vi "Cycling_No_DAQ_Tasks_All_3_PS_RT.vi"() -> ()   [LabVIEW 2020]
uses:
  <instrlib>/NH Research Regenerative Test Series/Public/Configure/Output Safety.ctl
panel:
  in  "PS error in 7":errorcluster caption="PS error in    (no error)"
  out "PS Visa Out 7":refnum<visa-resource-name>
  out "PS error out 7":errorcluster
  in  "PS error in 6":errorcluster caption="PS error in    (no error)"
  out "PS Visa Out 6":refnum<visa-resource-name>
  out "PS error out 6":errorcluster
  in  "PS error in 5":errorcluster caption="PS error in    (no error)"
  out "PS Visa Out 5":refnum<visa-resource-name>
  out "PS error out 5":errorcluster
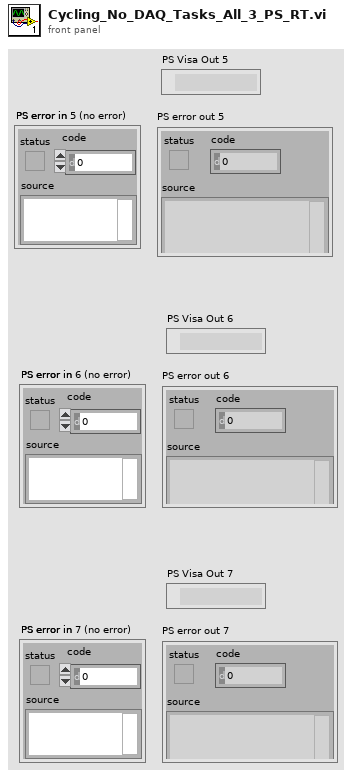
[diagram p1: front panel]
types:
  T1 = enum16{"\"30Q\"", "\"40T\"", "\"2P30Q\"", "\"3P30Q\"", "\"Nissan Leaf\"", ""}
  T2 = typedef "Output Safety.ctl" = cluster{"Min Voltage (V)":dbl, "Min Voltage Time (s)":dbl, "Max Voltage (V)":dbl, "Max Voltage Time (s)":dbl, "Max Sink Current (A)":dbl, "Max Sink Current Time (s)":dbl, "Max Source Current (A)":dbl, "Max Source Current Time (s)":dbl, "Max Sink Power (W)":dbl, "Max Sink Power Time (s)":dbl, "Max Source Power (W)":dbl, "Max Source Power Time (s)":dbl}
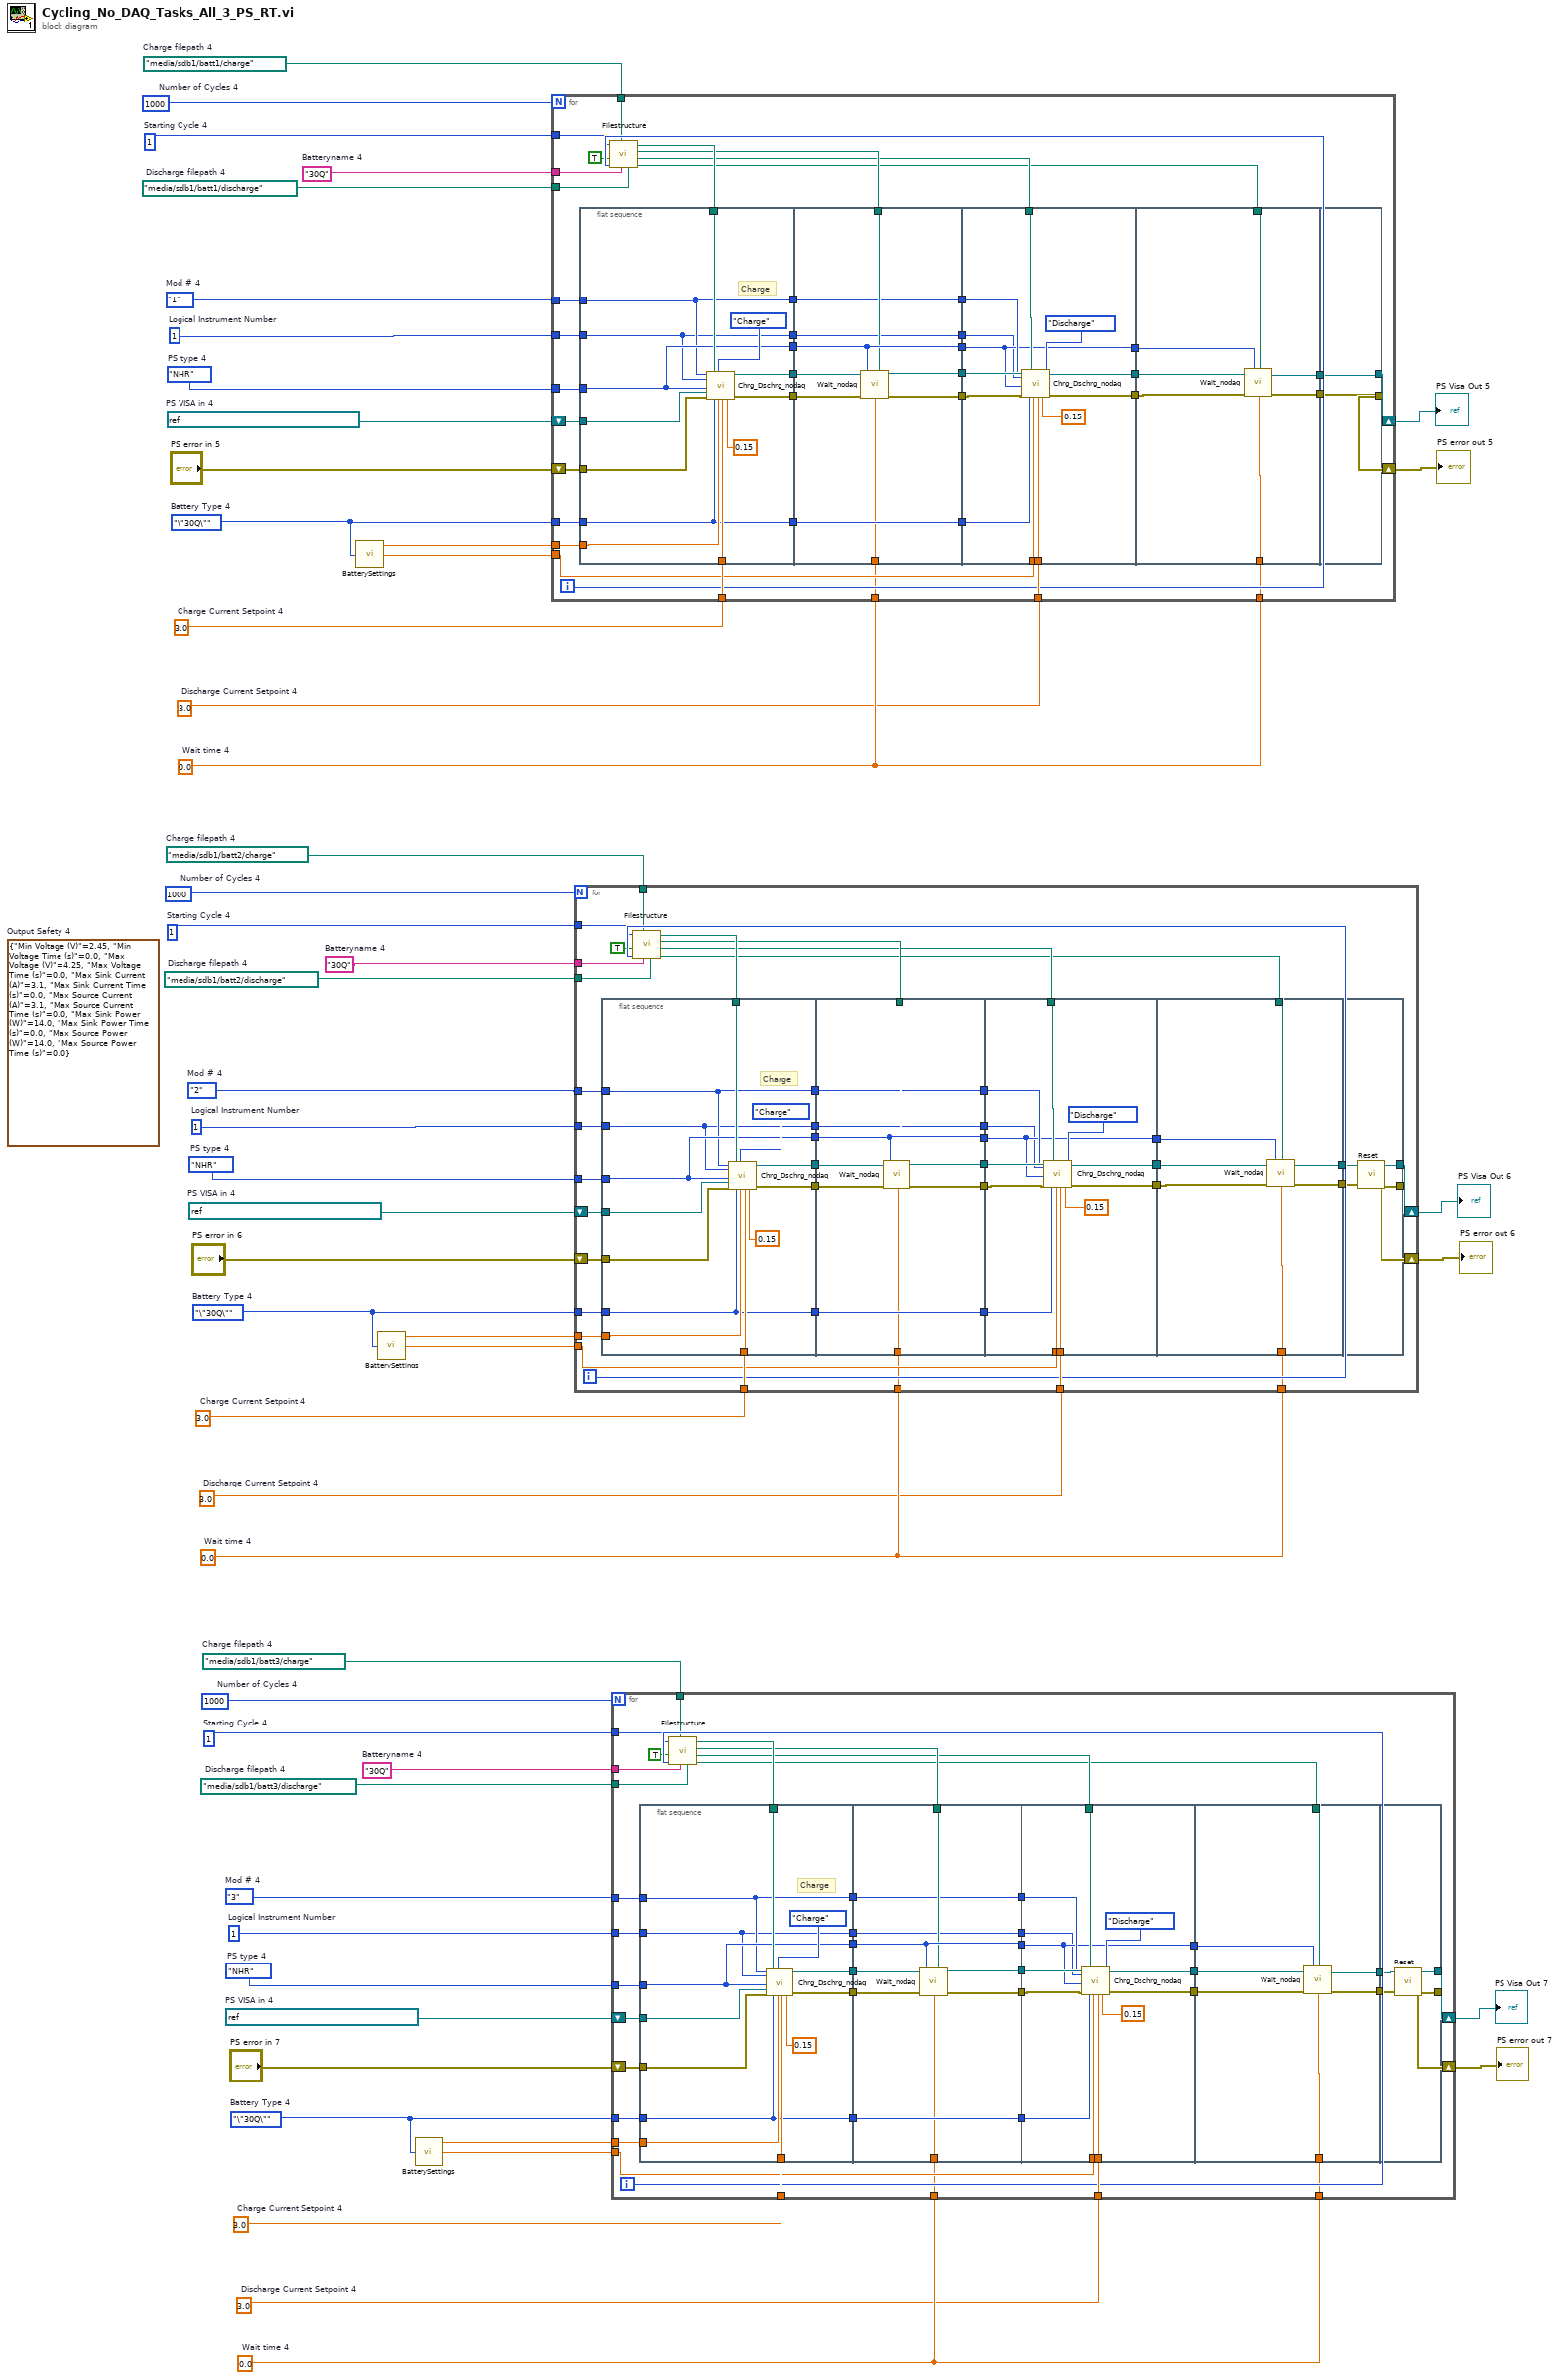
[diagram p0: block diagram]
diagram:
  w1 = u32 1  # Logical Instrument Number
  w3 = 1000  # Number of Cycles 4
  w4 = 1  # Starting Cycle 4
  w2 = path "/media/sdb1/batt3/charge"  # Charge filepath 4
  w5 = "30Q"  # Batteryname 4
  w6 = path "/media/sdb1/batt3/discharge"  # Discharge filepath 4
  w8 = enum16{"ITECH", "NHR"}."NHR"  # PS type 4
  w16 = 0.0  # Wait time 4
  w15 = 3.0  # Discharge Current Setpoint 4
  w14 = 3.0  # Charge Current Setpoint 4
  w11 = T1."\"30Q\""  # Battery Type 4
  w9 = refnum<visa-resource-name> "TCPIP0::192.168.0.94::inst0::INSTR"  # PS VISA in 4
  w7 = enum16{"0", "1", "2", "3"}."3"  # Mod # 4
  w19 = u32 1  # Logical Instrument Number
  w21 = 1000  # Number of Cycles 4
  w22 = 1  # Starting Cycle 4
  w20 = path "/media/sdb1/batt2/charge"  # Charge filepath 4
  w23 = "30Q"  # Batteryname 4
  w24 = path "/media/sdb1/batt2/discharge"  # Discharge filepath 4
  (unwired) T2 {"Min Voltage (V)"=2.45, "Min Voltage Time (s)"=0.0, "Max Voltage (V)"=4.25, "Max Voltage Time (s)"=0.0, "Max Sink Current (A)"=3.1, "Max Sink Current Time (s)"=0.0, "Max Source Current (A)"=3.1, "Max Source Current Time (s)"=0.0, "Max Sink Power (W)"=14.0, "Max Sink Power Time (s)"=0.0, "Max Source Power (W)"=14.0, "Max Source Power Time (s)"=0.0}  # Output Safety 4
  w26 = enum16{"ITECH", "NHR"}."NHR"  # PS type 4
  w34 = 0.0  # Wait time 4
  w33 = 3.0  # Discharge Current Setpoint 4
  w32 = 3.0  # Charge Current Setpoint 4
  w29 = T1."\"30Q\""  # Battery Type 4
  w27 = refnum<visa-resource-name> "TCPIP0::192.168.0.93::inst0::INSTR"  # PS VISA in 4
  w25 = enum16{"0", "1", "2", "3"}."2"  # Mod # 4
  w37 = u32 1  # Logical Instrument Number
  w39 = 1000  # Number of Cycles 4
  w40 = 1  # Starting Cycle 4
  w38 = path "/media/sdb1/batt1/charge"  # Charge filepath 4
  w41 = "30Q"  # Batteryname 4
  w42 = path "/media/sdb1/batt1/discharge"  # Discharge filepath 4
  w44 = enum16{"ITECH", "NHR"}."NHR"  # PS type 4
  w52 = 0.0  # Wait time 4
  w51 = 3.0  # Discharge Current Setpoint 4
  w50 = 3.0  # Charge Current Setpoint 4
  w47 = T1."\"30Q\""  # Battery Type 4
  w45 = refnum<visa-resource-name> "TCPIP0::192.168.0.92::inst0::INSTR"  # PS VISA in 4
  w43 = enum16{"0", "1", "2", "3"}."1"  # Mod # 4
  n1 = call "BatterySettings.vi"("Battery Type"=w47) -> ("Min Voltage (V)"=w49:dbl, "Max Voltage (V)"=w48:dbl)  [unwired: 2 in, 1 out]
  n2 = call "BatterySettings.vi"("Battery Type"=w29) -> ("Min Voltage (V)"=w31:dbl, "Max Voltage (V)"=w30:dbl)  [unwired: 2 in, 1 out]
  n3 = call "BatterySettings.vi"("Battery Type"=w11) -> ("Min Voltage (V)"=w13:dbl, "Max Voltage (V)"=w12:dbl)  [unwired: 2 in, 1 out]
  n4 = for {
    N: w39 -> [_]
    tunnel: w44 -> [w86]
    tunnel: w48 -> [w83]
    tunnel: w47 -> [w82]
    tunnel: w50 -> [w81]
    tunnel: w49 -> [w80]
    tunnel: w51 -> [w79]
    shift-right: [w73] -> w53
    shift-left: w45 -> [w85]
    shift-right: [w74] -> w54
    shift-left: "PS error in 5" -> [w84]
    tunnel: w40 -> [w71]
    tunnel: w41 -> [w69]
    tunnel: w42 -> [w68]
    tunnel: w38 -> [w67]
    tunnel: w52 -> [w62]
    tunnel: w52 -> [w61]
    tunnel: w43 -> [w60]
    tunnel: w37 -> [w57]
    i -> [w72]
    n5 = flat-sequence {
      tunnel: w86 -> [w98]
      tunnel: w85 -> [w100]
      tunnel: w84 -> [w101]
      tunnel: w82 -> [w99]
      tunnel: w83 -> [w102]
      tunnel: w81 -> [w103]
      tunnel: [w98] -> w95
      tunnel: [w99] -> w94
      tunnel: w78 -> [w108]
      tunnel: [w106] -> w64
      tunnel: [w105] -> w63
      tunnel: w60 -> [w97]
      tunnel: [w97] -> w58
      tunnel: w57 -> [w96]
      tunnel: [w96] -> w56
      tunnel: w95 -> [w117]
      tunnel: [w114] -> w93
      tunnel: [w115] -> w92
      tunnel: [w117] -> w91
      tunnel: w94 -> [w118]
      tunnel: [w118] -> w90
      tunnel: w77 -> [w116]
      tunnel: w64 -> [w113]
      tunnel: w63 -> [w112]
      tunnel: w61 -> [w111]
      tunnel: [w110] -> w59
      tunnel: w58 -> [w110]
      tunnel: w56 -> [w109]
      tunnel: [w109] -> w55
      tunnel: w93 -> [w127]
      tunnel: w92 -> [w128]
      tunnel: w91 -> [w121]
      tunnel: w90 -> [w130]
      tunnel: w80 -> [w129]
      tunnel: w79 -> [w120]
      tunnel: w76 -> [w126]
      tunnel: [w123] -> w89
      tunnel: [w124] -> w88
      tunnel: [w121] -> w87
      tunnel: w59 -> [w122]
      tunnel: w55 -> [w119]
      tunnel: w75 -> [w137]
      tunnel: w89 -> [w138]
      tunnel: w88 -> [w135]
      tunnel: w87 -> [w133]
      tunnel: [w136] -> w66
      tunnel: [w134] -> w65
      tunnel: w62 -> [w132]
      tunnel: [w140] -> w73
      tunnel: [w139] -> w74
      tunnel: w66 -> [w139]
      tunnel: w65 -> [w140]
      frame #0 {
        # "Charge"
        n6 = call "Chrg_Dschrg_nodaq.vi"("Mod #"=w97, "Logical Instrument Number"=w96, "PS type"=w98, "PS VISA in"=w100, "PS error in"=w101, "CyclePath"=w108, "Battery Type"=w99, "Charge/discharge"=enum8{"Charge", "Discharge"}."Charge", "Charge/Discharge Voltage Setpoint"=w102, "Current Setpoint"=w103, "Current Cutoff"=0.15) -> ("PS VISA out"=w106:refnum<visa-resource-name>, "PS error out"=w105:errorcluster)  [unwired: 7 in]
      }
      frame #1 {
        n7 = call "Wait_nodaq.vi"("PS type"=w117, "PS VISA in"=w113, "PS error in"=w112, "Wait Filepath"=w116, "Wait time"=w111) -> ("PS Visa Out"=w114:refnum<visa-resource-name>, "PS error out"=w115:errorcluster)  [unwired: 9 in]
      }
      frame #2 {
        n8 = call "Chrg_Dschrg_nodaq.vi"("Mod #"=w122, "Logical Instrument Number"=w119, "PS type"=w121, "PS VISA in"=w127, "PS error in"=w128, "CyclePath"=w126, "Battery Type"=w130, "Charge/discharge"=enum8{"Charge", "Discharge"}."Discharge", "Charge/Discharge Voltage Setpoint"=w129, "Current Setpoint"=w120, "Current Cutoff"=0.15) -> ("PS VISA out"=w123:refnum<visa-resource-name>, "PS error out"=w124:errorcluster)  [unwired: 7 in]
      }
      frame #3 {
        n9 = call "Wait_nodaq.vi"("PS type"=w133, "PS VISA in"=w138, "PS error in"=w135, "Wait Filepath"=w137, "Wait time"=w132) -> ("PS Visa Out"=w134:refnum<visa-resource-name>, "PS error out"=w136:errorcluster)  [unwired: 9 in]
      }
      frame #4 {
      }
    }
    n10 = call "Filestructure.vi"("Discharge filepath"=w68, "Batteryname"=w69, "Charge filepath"=w67, "For loop i"=w72, "In for loop"=TRUE, "Starting Cycle"=w71) -> ("DischargeWaitPath"=w75:path, "DischargeCyclePath"=w76:path, "ChargeWaitPath"=w77:path, "ChargeCyclePath"=w78:path)  [unwired: 1 in, 1 out]
  }
  "PS error out 5" <- w54
  "PS Visa Out 5" <- w53
  n11 = for {
    N: w21 -> [_]
    tunnel: w26 -> [w172]
    tunnel: w30 -> [w169]
    tunnel: w29 -> [w168]
    tunnel: w32 -> [w167]
    tunnel: w31 -> [w166]
    tunnel: w33 -> [w165]
    shift-right: [w159] -> w35
    shift-left: w27 -> [w171]
    shift-right: [w160] -> w36
    shift-left: "PS error in 6" -> [w170]
    tunnel: w22 -> [w157]
    tunnel: w23 -> [w155]
    tunnel: w24 -> [w154]
    tunnel: w20 -> [w153]
    tunnel: w34 -> [w148]
    tunnel: w34 -> [w147]
    tunnel: w25 -> [w146]
    tunnel: w19 -> [w143]
    i -> [w158]
    n12 = flat-sequence {
      tunnel: w172 -> [w184]
      tunnel: w171 -> [w186]
      tunnel: w170 -> [w187]
      tunnel: w168 -> [w185]
      tunnel: w169 -> [w188]
      tunnel: w167 -> [w189]
      tunnel: [w184] -> w181
      tunnel: [w185] -> w180
      tunnel: w164 -> [w194]
      tunnel: [w192] -> w150
      tunnel: [w191] -> w149
      tunnel: w146 -> [w183]
      tunnel: [w183] -> w144
      tunnel: w143 -> [w182]
      tunnel: [w182] -> w142
      tunnel: w181 -> [w203]
      tunnel: [w200] -> w179
      tunnel: [w201] -> w178
      tunnel: [w203] -> w177
      tunnel: w180 -> [w204]
      tunnel: [w204] -> w176
      tunnel: w163 -> [w202]
      tunnel: w150 -> [w199]
      tunnel: w149 -> [w198]
      tunnel: w147 -> [w197]
      tunnel: [w196] -> w145
      tunnel: w144 -> [w196]
      tunnel: w142 -> [w195]
      tunnel: [w195] -> w141
      tunnel: w179 -> [w213]
      tunnel: w178 -> [w214]
      tunnel: w177 -> [w207]
      tunnel: w176 -> [w216]
      tunnel: w166 -> [w215]
      tunnel: w165 -> [w206]
      tunnel: w162 -> [w212]
      tunnel: [w209] -> w175
      tunnel: [w210] -> w174
      tunnel: [w207] -> w173
      tunnel: w145 -> [w208]
      tunnel: w141 -> [w205]
      tunnel: w161 -> [w223]
      tunnel: w175 -> [w224]
      tunnel: w174 -> [w221]
      tunnel: w173 -> [w219]
      tunnel: [w222] -> w152
      tunnel: [w220] -> w151
      tunnel: w148 -> [w218]
      tunnel: [w227] -> w159
      tunnel: [w225] -> w160
      tunnel: w152 -> [w226]
      tunnel: w151 -> [w228]
      frame #0 {
        # "Charge"
        n13 = call "Chrg_Dschrg_nodaq.vi"("Mod #"=w183, "Logical Instrument Number"=w182, "PS type"=w184, "PS VISA in"=w186, "PS error in"=w187, "CyclePath"=w194, "Battery Type"=w185, "Charge/discharge"=enum8{"Charge", "Discharge"}."Charge", "Charge/Discharge Voltage Setpoint"=w188, "Current Setpoint"=w189, "Current Cutoff"=0.15) -> ("PS VISA out"=w192:refnum<visa-resource-name>, "PS error out"=w191:errorcluster)  [unwired: 7 in]
      }
      frame #1 {
        n14 = call "Wait_nodaq.vi"("PS type"=w203, "PS VISA in"=w199, "PS error in"=w198, "Wait Filepath"=w202, "Wait time"=w197) -> ("PS Visa Out"=w200:refnum<visa-resource-name>, "PS error out"=w201:errorcluster)  [unwired: 9 in]
      }
      frame #2 {
        n15 = call "Chrg_Dschrg_nodaq.vi"("Mod #"=w208, "Logical Instrument Number"=w205, "PS type"=w207, "PS VISA in"=w213, "PS error in"=w214, "CyclePath"=w212, "Battery Type"=w216, "Charge/discharge"=enum8{"Charge", "Discharge"}."Discharge", "Charge/Discharge Voltage Setpoint"=w215, "Current Setpoint"=w206, "Current Cutoff"=0.15) -> ("PS VISA out"=w209:refnum<visa-resource-name>, "PS error out"=w210:errorcluster)  [unwired: 7 in]
      }
      frame #3 {
        n16 = call "Wait_nodaq.vi"("PS type"=w219, "PS VISA in"=w224, "PS error in"=w221, "Wait Filepath"=w223, "Wait time"=w218) -> ("PS Visa Out"=w220:refnum<visa-resource-name>, "PS error out"=w222:errorcluster)  [unwired: 9 in]
      }
      frame #4 {
        n17 = call "Reset.vi"("error in"=w226, "VISA resource name"=w228) -> ("error out"=w225:errorcluster, "VISA resource name out"=w227:refnum<visa-resource-name>)  [unwired: 8 in]
      }
    }
    n18 = call "Filestructure.vi"("Discharge filepath"=w154, "Batteryname"=w155, "Charge filepath"=w153, "For loop i"=w158, "In for loop"=TRUE, "Starting Cycle"=w157) -> ("DischargeWaitPath"=w161:path, "DischargeCyclePath"=w162:path, "ChargeWaitPath"=w163:path, "ChargeCyclePath"=w164:path)  [unwired: 1 in, 1 out]
  }
  "PS error out 6" <- w36
  "PS Visa Out 6" <- w35
  n19 = for {
    N: w3 -> [_]
    tunnel: w8 -> [w260]
    tunnel: w12 -> [w257]
    tunnel: w11 -> [w256]
    tunnel: w14 -> [w255]
    tunnel: w13 -> [w254]
    tunnel: w15 -> [w253]
    shift-right: [w247] -> w17
    shift-left: w9 -> [w259]
    shift-right: [w248] -> w18
    shift-left: "PS error in 7" -> [w258]
    tunnel: w4 -> [w245]
    tunnel: w5 -> [w243]
    tunnel: w6 -> [w242]
    tunnel: w2 -> [w241]
    tunnel: w16 -> [w236]
    tunnel: w16 -> [w235]
    tunnel: w7 -> [w234]
    tunnel: w1 -> [w231]
    i -> [w246]
    n20 = flat-sequence {
      tunnel: w260 -> [w272]
      tunnel: w259 -> [w274]
      tunnel: w258 -> [w275]
      tunnel: w256 -> [w273]
      tunnel: w257 -> [w276]
      tunnel: w255 -> [w277]
      tunnel: [w272] -> w269
      tunnel: [w273] -> w268
      tunnel: w252 -> [w282]
      tunnel: [w280] -> w238
      tunnel: [w279] -> w237
      tunnel: w234 -> [w271]
      tunnel: [w271] -> w232
      tunnel: w231 -> [w270]
      tunnel: [w270] -> w230
      tunnel: w269 -> [w291]
      tunnel: [w288] -> w267
      tunnel: [w289] -> w266
      tunnel: [w291] -> w265
      tunnel: w268 -> [w292]
      tunnel: [w292] -> w264
      tunnel: w251 -> [w290]
      tunnel: w238 -> [w287]
      tunnel: w237 -> [w286]
      tunnel: w235 -> [w285]
      tunnel: [w284] -> w233
      tunnel: w232 -> [w284]
      tunnel: w230 -> [w283]
      tunnel: [w283] -> w229
      tunnel: w267 -> [w301]
      tunnel: w266 -> [w302]
      tunnel: w265 -> [w295]
      tunnel: w264 -> [w304]
      tunnel: w254 -> [w303]
      tunnel: w253 -> [w294]
      tunnel: w250 -> [w300]
      tunnel: [w297] -> w263
      tunnel: [w298] -> w262
      tunnel: [w295] -> w261
      tunnel: w233 -> [w296]
      tunnel: w229 -> [w293]
      tunnel: w249 -> [w311]
      tunnel: w263 -> [w312]
      tunnel: w262 -> [w309]
      tunnel: w261 -> [w307]
      tunnel: [w310] -> w240
      tunnel: [w308] -> w239
      tunnel: w236 -> [w306]
      tunnel: [w315] -> w247
      tunnel: [w313] -> w248
      tunnel: w240 -> [w314]
      tunnel: w239 -> [w316]
      frame #0 {
        # "Charge"
        n21 = call "Chrg_Dschrg_nodaq.vi"("Mod #"=w271, "Logical Instrument Number"=w270, "PS type"=w272, "PS VISA in"=w274, "PS error in"=w275, "CyclePath"=w282, "Battery Type"=w273, "Charge/discharge"=enum8{"Charge", "Discharge"}."Charge", "Charge/Discharge Voltage Setpoint"=w276, "Current Setpoint"=w277, "Current Cutoff"=0.15) -> ("PS VISA out"=w280:refnum<visa-resource-name>, "PS error out"=w279:errorcluster)  [unwired: 7 in]
      }
      frame #1 {
        n22 = call "Wait_nodaq.vi"("PS type"=w291, "PS VISA in"=w287, "PS error in"=w286, "Wait Filepath"=w290, "Wait time"=w285) -> ("PS Visa Out"=w288:refnum<visa-resource-name>, "PS error out"=w289:errorcluster)  [unwired: 9 in]
      }
      frame #2 {
        n23 = call "Chrg_Dschrg_nodaq.vi"("Mod #"=w296, "Logical Instrument Number"=w293, "PS type"=w295, "PS VISA in"=w301, "PS error in"=w302, "CyclePath"=w300, "Battery Type"=w304, "Charge/discharge"=enum8{"Charge", "Discharge"}."Discharge", "Charge/Discharge Voltage Setpoint"=w303, "Current Setpoint"=w294, "Current Cutoff"=0.15) -> ("PS VISA out"=w297:refnum<visa-resource-name>, "PS error out"=w298:errorcluster)  [unwired: 7 in]
      }
      frame #3 {
        n24 = call "Wait_nodaq.vi"("PS type"=w307, "PS VISA in"=w312, "PS error in"=w309, "Wait Filepath"=w311, "Wait time"=w306) -> ("PS Visa Out"=w308:refnum<visa-resource-name>, "PS error out"=w310:errorcluster)  [unwired: 9 in]
      }
      frame #4 {
        n25 = call "Reset.vi"("error in"=w314, "VISA resource name"=w316) -> ("error out"=w313:errorcluster, "VISA resource name out"=w315:refnum<visa-resource-name>)  [unwired: 8 in]
      }
    }
    n26 = call "Filestructure.vi"("Discharge filepath"=w242, "Batteryname"=w243, "Charge filepath"=w241, "For loop i"=w246, "In for loop"=TRUE, "Starting Cycle"=w245) -> ("DischargeWaitPath"=w249:path, "DischargeCyclePath"=w250:path, "ChargeWaitPath"=w251:path, "ChargeCyclePath"=w252:path)  [unwired: 1 in, 1 out]
  }
  "PS error out 7" <- w18
  "PS Visa Out 7" <- w17
